vi "RSZVB Calibration Manager.vi"(7 "File Name (D:\\user\\data)":string="D:\\user\\data", 8 "error in (no error)":errorcluster {"code" format="%.0x"}, 9 "Operation to be Performed (0: Copy)":i32(ring) items=["Copy", "Apply", "Resolve Pool Link", "Delete", "Apply to All Channels", "Resolve Pool Link For All Channels", "Merge"], 10 "Channel (1)":i32=1, 11 "VISA session":refnum<visa-resource-name>) -> (0 "error out":errorcluster {"code" format="%.0x"}, 3 "dup VISA session":refnum<visa-resource-name>)   [LabVIEW 2011]
doc: "This VI provides operations which allows to store system error correction data to the cal pool and to assign stored correction data to channels:\n\n Copy\n Apply\n Resolve Pool Link\n Delete\n\nRemote-control command(s):\nMMEMory:STORe:CORRection <Ch>,'<file_name>'\nMMEMory:LOAD:CORRection <Ch>,'<file_name>'\nMMEMory:LOAD:CORRection:RESolve <Ch>,'<file_name>'\nMMEMory:DELete:CORRection '<file_name>'"
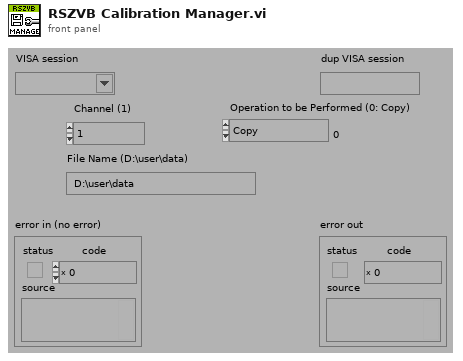
[diagram p1: front panel]
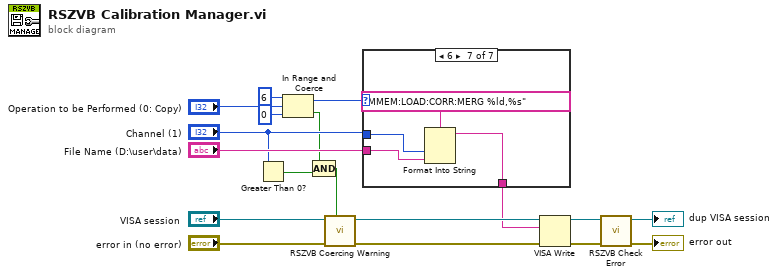
[diagram p0: block diagram]
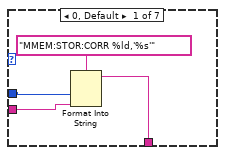
[diagram p2: hidden frame]
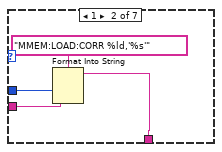
[diagram p3: hidden frame]
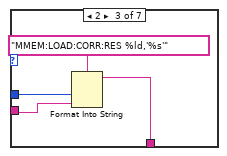
[diagram p4: hidden frame]
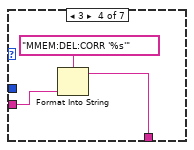
[diagram p5: hidden frame]
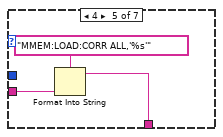
[diagram p6: hidden frame]
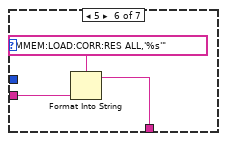
[diagram p7: hidden frame]
diagram:
  n1 = Greater Than 0?(x="Channel (1)") -> (x > 0?=w3:bool)
  n2 = In Range and Coerce(upper limit=6, x="Operation to be Performed (0: Copy)", lower limit=0) -> (coerced(x)=w16:i32, In Range?=w2:bool)
  n3 = Compound Arithmetic op=AND(w2, w3) -> (w1:bool)
  n4 = call "RSZVB Coercing Warning.vi"("In Range?"=w1, "error in (no error)"="error in (no error)", "VISA session"="VISA session") -> ("error out"=w13:errorcluster, "dup VISA session"=w12:refnum<visa-resource-name>)  [unwired: 7 in]
  n5 = case shown="6" w16 {
    tunnel: [w21 w25 w28 w32 w35 w38 w40] -> w11
    tunnel: "Channel (1)" -> [w20 w23 w29 _ _ _ w42]
    tunnel: "File Name (D:\\user\\data)" -> [w19 w24 w27 w31 w34 w37 w41]
    frame 0, Default {
      n6 = Format Into String(format string="MMEM:STOR:CORR %ld,'%s'", w20, w19) -> (resulting string=w21:string)  [unwired: 2 in, 1 out]
    }
    frame 1 {
      n7 = Format Into String(format string="MMEM:LOAD:CORR %ld,'%s'", w23, w24) -> (resulting string=w25:string)  [unwired: 2 in, 1 out]
    }
    frame 2 {
      n8 = Format Into String(format string="MMEM:LOAD:CORR:RES %ld,'%s'", w29, w27) -> (resulting string=w28:string)  [unwired: 2 in, 1 out]
    }
    frame 3 {
      n9 = Format Into String(format string="MMEM:DEL:CORR '%s'", w31) -> (resulting string=w32:string)  [unwired: 2 in, 1 out]
    }
    frame 4 {
      n10 = Format Into String(format string="MMEM:LOAD:CORR ALL,'%s'", w34) -> (resulting string=w35:string)  [unwired: 2 in, 1 out]
    }
    frame 5 {
      n11 = Format Into String(format string="MMEM:LOAD:CORR:RES ALL,'%s'", w37) -> (resulting string=w38:string)  [unwired: 2 in, 1 out]
    }
    frame 6 {
      n12 = Format Into String(format string="MMEM:LOAD:CORR:MERG %ld,%s", w42, w41) -> (resulting string=w40:string)  [unwired: 2 in, 1 out]
    }
  }
  n13 = VISA Write(VISA resource name=w12, write buffer=w11, error in (no error)=w13) -> (VISA resource name out=w15:refnum<visa-resource-name>, error out=w14:errorcluster)  [unwired: 1 out]
  n14 = call "RSZVB Check Error.vi"("error in (no error)"=w14, "VISA session"=w15) -> ("error out"=→"error out":errorcluster, "dup VISA session"=→"dup VISA session":refnum<visa-resource-name>)  [unwired: 8 in]
